vi "Config_3457_Norm.vi"(8 "error in (no error)":errorcluster) -> (0 "error out":errorcluster)   [LabVIEW 2020]
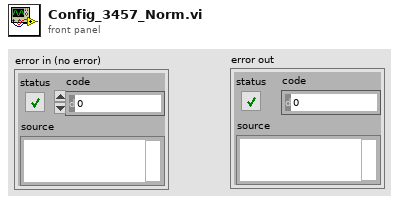
[diagram p1: front panel]
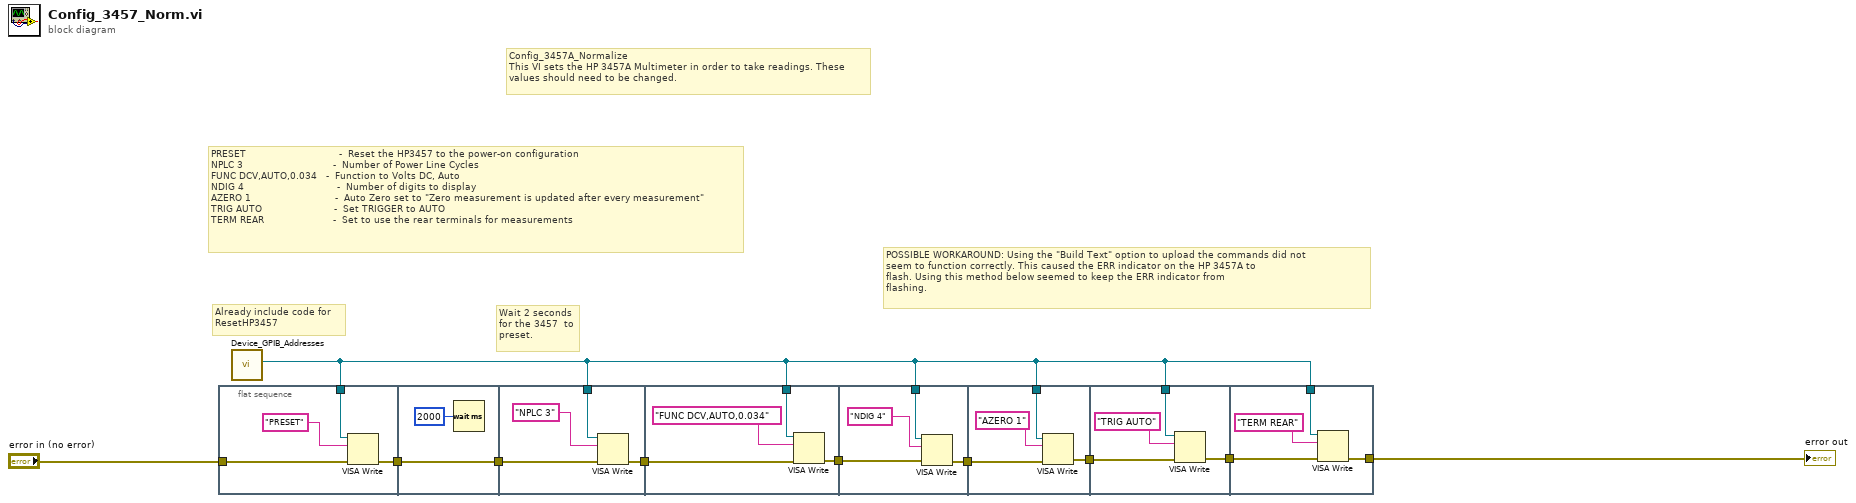
[diagram p0: block diagram]
diagram:
  # "Already include code for\nResetHP3457"
  # "Config_3457A_Normalize\nThis VI sets the HP 3457A Multimeter in order to take readings. These\nvalues should need to be changed."
  # "Wait 2 seconds\nfor the 3457  to\npreset."
  # "POSSIBLE WORKAROUND: Using the \"Build Text\" option to upload the commands did not\nseem to function correctly. This caused the ERR indicator on the HP 3457A to\nflash. Using this method below seemed to keep the ERR indicator from\nflashing."
  # "PRESET                               -  Reset the HP3457 to the power-on configuration\nNPLC 3                              -  Number of Power Line Cycles\nFUNC DCV,AUTO,0.034   -  Function to Volts DC, Auto \nNDIG 4                               -  Number of digits to display\nAZERO 1                            -  Auto Zero set to \"Zero measurement is updated after every measurement\"\nTRIG AUTO                        -  Set TRIGGER to AUTO\nTERM REAR                       -  Set to use the rear terminals for measurements"
  n1 = flat-sequence {
    tunnel: "error in (no error)" -> [w13]
    tunnel: [w12] -> w2
    tunnel: w1 -> [w11]
    tunnel: [w15] -> w3
    tunnel: w2 -> [w15]
    tunnel: w1 -> [w20]
    tunnel: [w17] -> w10
    tunnel: w3 -> [w18]
    tunnel: w1 -> [w23]
    tunnel: w10 -> [w22]
    tunnel: [w21] -> w9
    tunnel: w9 -> [w28]
    tunnel: w1 -> [w26]
    tunnel: [w25] -> w8
    tunnel: w1 -> [w31]
    tunnel: w8 -> [w30]
    tunnel: [w29] -> w7
    tunnel: w7 -> [w36]
    tunnel: w1 -> [w35]
    tunnel: [w33] -> w6
    tunnel: w1 -> [w40]
    tunnel: w6 -> [w39]
    tunnel: [w37] -> w5
    frame #0 {
      n2 = VISA Write(VISA resource name=w11, write buffer="PRESET", error in (no error)=w13) -> (error out=w12:errorcluster)  [unwired: 2 out]
    }
    frame #1 {
      n3 = Wait (ms)(milliseconds to wait=u32 2000) -> ()  [unwired: 1 out]
    }
    frame #2 {
      n4 = VISA Write(VISA resource name=w20, write buffer="NPLC 3", error in (no error)=w18) -> (error out=w17:errorcluster)  [unwired: 2 out]
    }
    frame #3 {
      n5 = VISA Write(VISA resource name=w23, write buffer="FUNC DCV,AUTO,0.034", error in (no error)=w22) -> (error out=w21:errorcluster)  [unwired: 2 out]
    }
    frame #4 {
      n6 = VISA Write(VISA resource name=w26, write buffer="NDIG 4", error in (no error)=w28) -> (error out=w25:errorcluster)  [unwired: 2 out]
    }
    frame #5 {
      n7 = VISA Write(VISA resource name=w31, write buffer="AZERO 1", error in (no error)=w30) -> (error out=w29:errorcluster)  [unwired: 2 out]
    }
    frame #6 {
      n8 = VISA Write(VISA resource name=w35, write buffer="TRIG AUTO", error in (no error)=w36) -> (error out=w33:errorcluster)  [unwired: 2 out]
    }
    frame #7 {
      n9 = VISA Write(VISA resource name=w40, write buffer="TERM REAR", error in (no error)=w39) -> (error out=w37:errorcluster)  [unwired: 2 out]
    }
  }
  n10 = call "Device_GPIB_Addresses.vi"() -> ("HP 3457A Address"=w1:refnum<visa-resource-name>)  [unwired: 9 in, 2 out]
  "error out" <- w5
